vi "FPGA_AIERRInvalidAccumulatorChannel.vi"(1 "error in (no error)":errorcluster) -> (0 "error out":errorcluster)   [LabVIEW 2017]
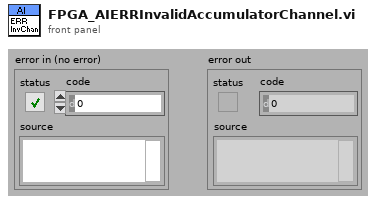
[diagram p1: front panel]
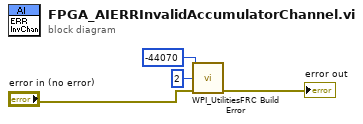
[diagram p0: block diagram]
diagram:
  n1 = call <vilib>:"WPI_UtilitiesFRC Build Error.vi"("error code"=-44070 ("code"), "chain levels to remove (1)"=2, "error in (no error)"="error in (no error)") -> ("error out"=→"error out":errorcluster)  [unwired: 2 in, 10 out]
